vi "Digital Output - Blink LED.vi"() -> ()   [LabVIEW 2015]
doc: "This example shows how to set an Arduino digital pin to an output, then toggle the voltage between low (0V) and high (5V) to drive an LED on and off."
uses:
  <vilib>/Aledyne-TSXperts/Arduino Compatible Compiler for LabVIEW/Code Generator/Arduino APIs/Digital/PinDirection.ctl
  <vilib>/Aledyne-TSXperts/Arduino Compatible Compiler for LabVIEW/Arduino Compatible Compiler for LabVIEW.lvlib
panel:
  in  "Digital Pin":u8=13
  # "Overview: Demonstrates how to toggle a digital pin on an Arduino to illuminate an LED.\n\nInstructions:\n1. Wire an LED's anode to a digital pin on the Arduino board and wire the cathode to a ground pin through a 220ohm or equivalent resistor (or use the onboard LED on pin 13).\n2. Set the Digital Pin wired below.\n3.  If this example has been loaded from the Arduino Compatible Compiler for LabVIEW, simply select Compile and Download.  Otherwise, open Tools>Arduino Compatible Compiler for LabVIEW in LabVIEW, then select File>Load VI, and select this VI and then Compile and Download.\n4. Observe the LED turning off and on."
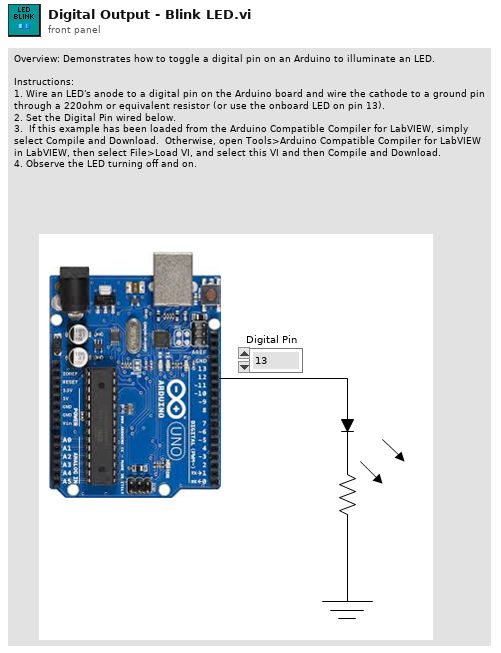
[diagram p1: front panel]
types:
  T1 = typedef "Arduino Compatible Compiler for LabVIEW.lvlib/PinDirection.ctl" = enum16{" INPUT", "OUTPUT", " INPUT_PULLUP"}
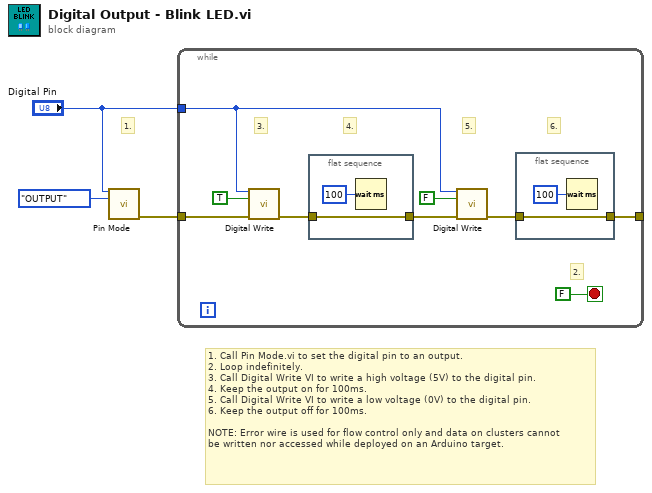
[diagram p0: block diagram]
diagram:
  # "1."
  # "1. Call Pin Mode.vi to set the digital pin to an output.\n2. Loop indefinitely.\n3. Call Digital Write VI to write a high voltage (5V) to the digital pin.\n4. Keep the output on for 100ms.\n5. Call Digital Write VI to write a low voltage (0V) to the digital pin.\n6. Keep the output off for 100ms.\n\nNOTE: Error wire is used for flow control only and data on clusters cannot\nbe written nor accessed while deployed on an Arduino target."
  n1 = call <vilib>:"Pin Mode.vi"("pin"="Digital Pin", "direction"=PinDirection."OUTPUT" ("Direction")) -> ("error out"=w3:errorcluster)  [unwired: 13 in]
  n2 = while {
    tunnel: "Digital Pin" -> [w9]
    tunnel: w3 -> [w8]
    tunnel: [w10] -> _
    stop <- FALSE stop-if-true
    # "2."
    # "6."
    # "5."
    # "4."
    # "3."
    n3 = call <vilib>:"Digital Write.vi"("pin"=w9, "state"=TRUE, "error in (no error)"=w8) -> ("error out"=w12:errorcluster)  [unwired: 12 in]
    n4 = flat-sequence {
      tunnel: [w15] -> w7
      tunnel: w12 -> [w15]
      frame #0 {
        n5 = Wait (ms)(milliseconds to wait=u32 100) -> ()  [unwired: 1 out]
      }
    }
    n6 = call <vilib>:"Digital Write.vi"("pin"=w9, "state"=FALSE, "error in (no error)"=w7) -> ("error out"=w11:errorcluster)  [unwired: 12 in]
    n7 = flat-sequence {
      tunnel: [w14] -> w10
      tunnel: w11 -> [w14]
      frame #0 {
        n8 = Wait (ms)(milliseconds to wait=u32 100) -> ()  [unwired: 1 out]
      }
    }
  }
